vi "VXM-MoveAbsolute.vi"(8 "error in (no error)":errorcluster, 9 "Move-Abs":T3 {"Polarization" items=["Vertical", "Horizontal"]}, 11 "Message que":T4) -> (0 "error out":errorcluster)   [LabVIEW 2018]
uses:
  Support/MessageQue/MessageQue.ctl
  Support/MessageQue/MessageCluster.ctl
  singleAxisMoveDef.ctl
  mmWaveAxis.ctl
  Support/MessageQue/MessageQue.lvlib
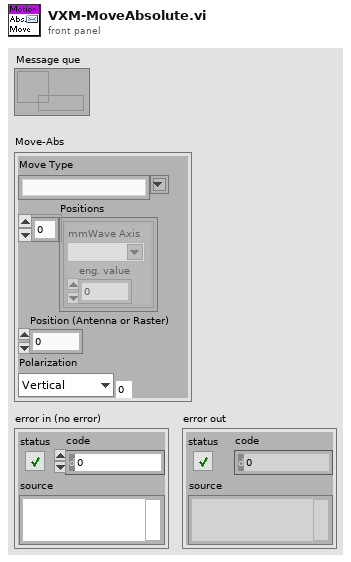
[diagram p1: front panel]
types:
  T1 = typedef "singleAxisMoveDef.ctl" = cluster{"mmWave Axis":T2, "eng. value":dbl}
  T2 = typedef "mmWaveAxis.ctl" = string
  T3 = cluster{"Move Type":string, "Positions":T1[], "Position (Antenna or Raster)":i32, "Polarization":u16}
  T4 = typedef "MessageQue.lvlib/MessageQue.ctl" = refnum<queue>
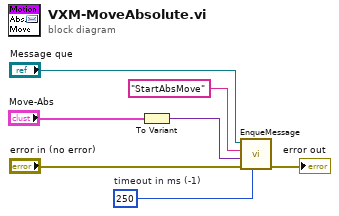
[diagram p0: block diagram]
diagram:
  w6 = 250  # timeout in ms (-1)
  n1 = To Variant(anything="Move-Abs") -> (Variant=w7:variant)
  n2 = call "EnqueMessage.vi"("timeout in ms (-1)"=w6, "error in"="error in (no error)", "Message Payload"=w7, "Message Command"="StartAbsMove", "Message que"="Message que") -> ("error out"=→"error out":errorcluster)  [unwired: 5 in, 1 out]
